vi "data_ref-waypt_0619.vi"() -> ()   [LabVIEW 2018]
panel:
  out "size 0619_testdrive R":i32
  out "size 0619_testdrive":i32
  out "0619_testdrive R":cluster{"X":dbl, "Y":dbl}[](graph)
  out "0619_testdrive":cluster{"X":dbl, "Y":dbl}[](graph)
  out "size ref waypt 0619 half F":i32
  out "크기":i32
  in  "dt2":u32
  in  "정지":bool
  out "XY 그래프 2":cluster{"X":dbl, "Y":dbl}[](graph)
  in  "길이":i32
  out "ref waypt 0619 half F":cluster{"X":dbl, "Y":dbl}[](graph)
  in  "dt":u32=1
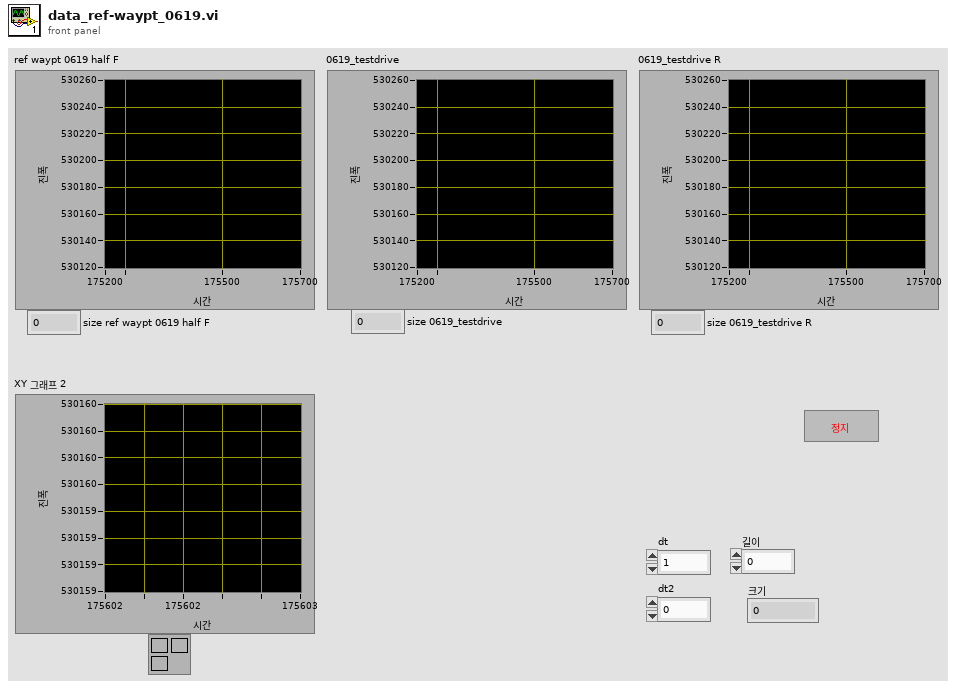
[diagram p1: front panel]
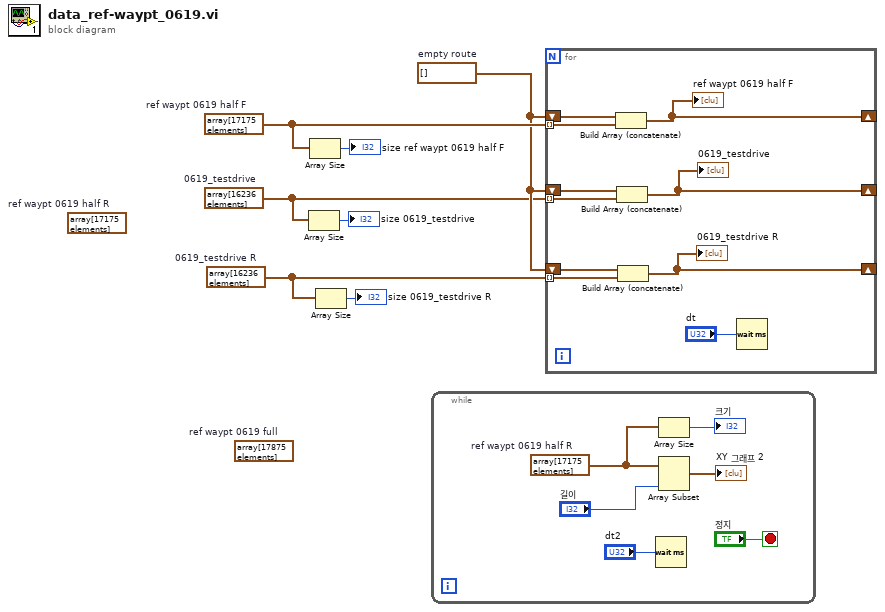
[diagram p0: block diagram]
diagram:
  w1 = cluster{"X":dbl, "Y":dbl}[] array[16236 elements]  # 0619_testdrive R
  w7 = cluster{"X":dbl, "Y":dbl}[] array[17175 elements]  # ref waypt 0619 half F
  (unwired) cluster{"X":dbl, "Y":dbl}[] array[17875 elements]  # ref waypt 0619 full
  w3 = cluster{dbl, dbl}[] array[16236 elements]  # 0619_testdrive
  w5 = cluster{"X":dbl, "Y":dbl}[] []  # empty route
  (unwired) cluster{"X":dbl, "Y":dbl}[] array[17175 elements]  # ref waypt 0619 half R
  n1 = Array Size(array=w3) -> (size(s)=→"size 0619_testdrive":i32)
  n2 = Array Size(array=w7) -> (size(s)=→"size ref waypt 0619 half F":i32)
  n3 = Array Size(array=w1) -> (size(s)=→"size 0619_testdrive R":i32)
  n4 = while {
    stop <- "정지" stop-if-true
    w8 = cluster{"X":dbl, "Y":dbl}[] array[17175 elements]  # ref waypt 0619 half R
    n5 = Wait (ms)(milliseconds to wait="dt2") -> ()  [unwired: 1 out]
    n6 = Array Size(array=w8) -> (size(s)=→"크기":i32)
    n7 = Array Subset(array=w8, length="길이") -> (→"XY 그래프 2":cluster{"X":dbl, "Y":dbl}[])  [unwired: 1 in]
  }
  n8 = for {
    shift-right: [w21] -> _
    shift-left: w5 -> [w23]
    tunnel: w7 -> [w20] mode=indexing
    shift-right: [w17] -> _
    shift-left: w5 -> [w19]
    tunnel: w3 -> [w18] mode=indexing
    shift-right: [w14] -> _
    shift-left: w5 -> [w16]
    tunnel: w1 -> [w15] mode=indexing
    n9 = Build Array (concatenate)(w23, w20) -> (w21:cluster{"X":dbl, "Y":dbl}[])
    "ref waypt 0619 half F" <- w21
    n10 = Build Array (concatenate)(w19, w18) -> (w17:cluster{"X":dbl, "Y":dbl}[])
    "0619_testdrive" <- w17
    n11 = Build Array (concatenate)(w16, w15) -> (w14:cluster{"X":dbl, "Y":dbl}[])
    "0619_testdrive R" <- w14
    n12 = Wait (ms)(milliseconds to wait="dt") -> ()  [unwired: 1 out]
  }
